vi "ICM Write Characters.vi"(8 "error in (no error)":errorcluster, 9 "Handle In":variant, 10 "Data In":string, 11 "OSDS Format":T1={"Data Stream Name"="", "Version"=0.0, "Author"="", "Reader Name"="", "Parser Name"="", "Description"="", "Comments"="", "Location"="", "Format String"="", "Frame Time"=0, "# of Channels"=0, "# of Records"=0, "Char/Record"=0, "Termination String\nor NTP IP"="", "Bus"=enum."Serial Port", "Port"=1, "Baud Rate"=9600, "Data Bits"=8, "Parity"=enum."None", "Stop Bits"=10, "Flow Control"=0, "Channel Names"=[], "Enabled"=[], "Initialization String"="", "Query String"="", "Reserved String"="", "Reserved Number"=0.0, "Date"=0.0, "Start Time"=0.0} {"Flow Control" items=["None", "XON/XOFF", "RTS/CTS", "XON/XOFF & RTS/CTS", "DTR/DSR", "XON/XOFF & DTR/DSR"]; "Stop Bits" items=["1.0"=10, "1.5"=15, "2.0"=20]; "Data Bits" min=5 max=8 step=1; "Start Time" format="%<%H:%M:%S>t"; "Date" format="%<%Y/%m/%d>T"; "Version" format="%.1g"}) -> (0 "error out":errorcluster, 2 "Bytes Written":i32)   [LabVIEW 2018]
doc: "OSDS Write Characters.vi\n\n This VI is used to write a frame of Siimulated or Play Back data to a communication port.\n\nOCC Streaming Data System Version 1.0\nJune, 2007 Original Code Consulting David Thomson\n www.originalcode.com"
uses:
  MICAS-X/Resources/OSDS/OSDS Subvis/OSDS Format.ctl
  MICAS-X/Resources/OSDS/OSDS Subvis/OSDS Bus.ctl
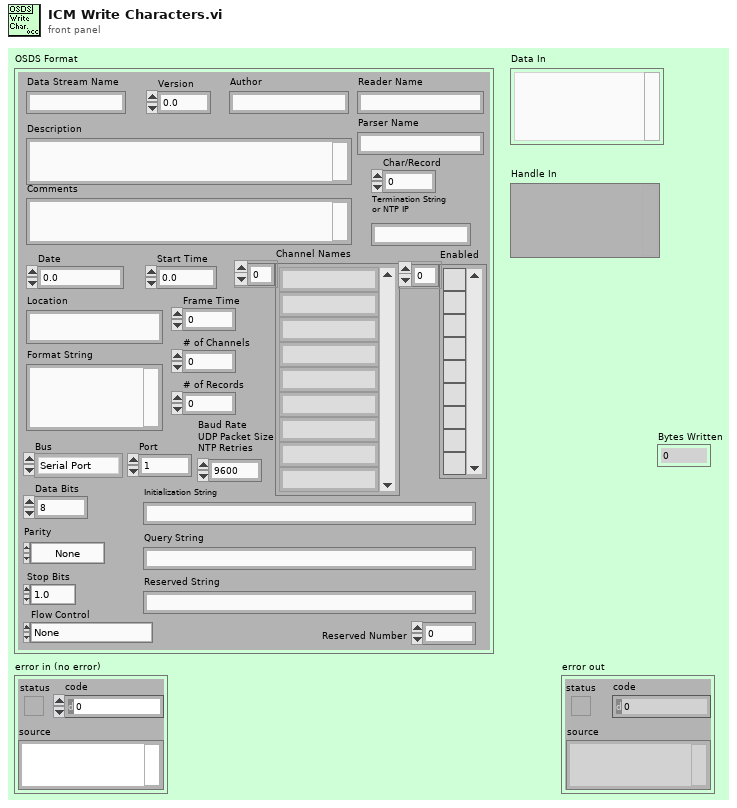
[diagram p1: front panel]
types:
  T1 = typedef "OSDS Format.ctl" = cluster{"Data Stream Name":string, "Version":sgl, "Author":string, "Reader Name":string, "Parser Name":string, "Description":string, "Comments":string, "Location":string, "Format String":string, "Frame Time":i32, "# of Channels":i32, "# of Records":i32, "Char/Record":i32, "Termination String\nor NTP IP":string, "Bus":T2, "Port":i32, "Baud Rate":u32, "Data Bits":u16, "Parity":enum16{"None", "Odd", "Even", "Mark", "Space"}, "Stop Bits":u16, "Flow Control":u16, "Channel Names":string[], "Enabled":bool[], "Initialization String":string, "Query String":string, "Reserved String":string, "Reserved Number":dbl, "Date":dbl, "Start Time":dbl}
  T2 = typedef "OSDS Bus.ctl" = enum16{"Serial Port", "UDP", "NTP", "Local Time", "UTC Time", "UDP MC", "TCP"}
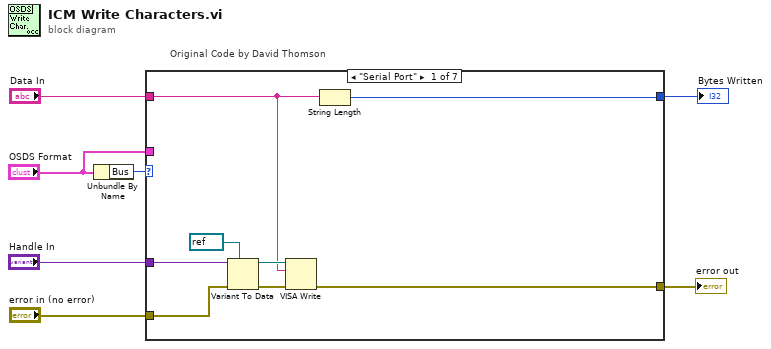
[diagram p0: block diagram]
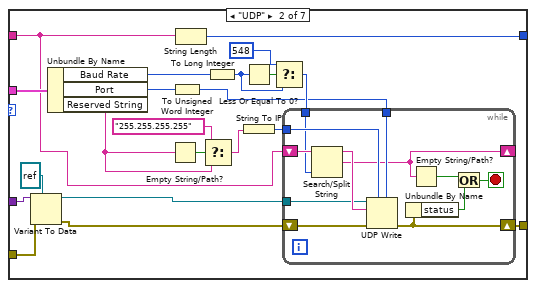
[diagram p2: hidden frame]
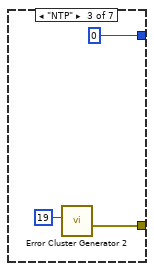
[diagram p3: hidden frame]
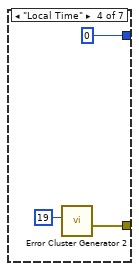
[diagram p4: hidden frame]
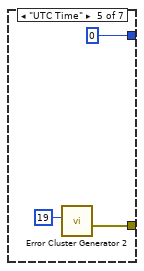
[diagram p5: hidden frame]
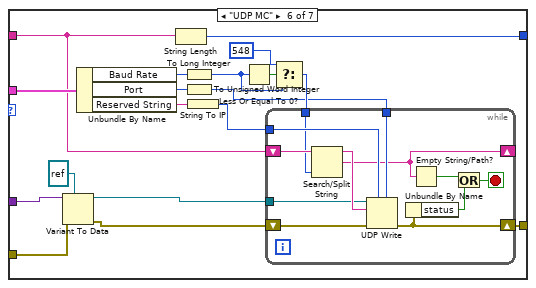
[diagram p6: hidden frame]
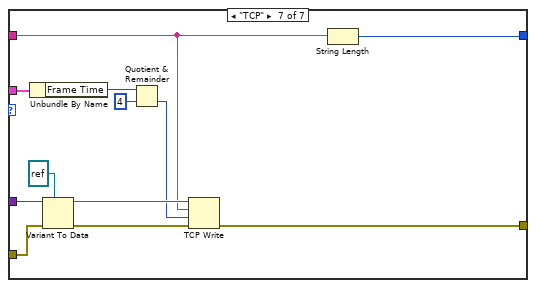
[diagram p7: hidden frame]
diagram:
  n1 = Unbundle By Name("OSDS Format") -> ("Bus"=w7:T2)
  n2 = case "Original Code by David Thomson" shown="\"Serial Port\"" w7 {
    tunnel: "Handle In" -> [w15 w36 _ _ _ w75 w99]
    tunnel: [w10 w28 w50 w52 w55 w67 w94] -> w5
    tunnel: "Data In" -> [w9 w18 _ _ _ w65 w93]
    tunnel: [w13 w34 0 0 0 w73 w92] -> w3
    tunnel: "OSDS Format" -> [_ w33 _ _ _ w72 w90]
    tunnel: "error in (no error)" -> [w8 w23 _ _ _ w61 w98]
    frame "Serial Port" {
      n3 = Variant To Data(error in=w8, type=refnum<visa-resource-name> refnum ("VISA resource name"), Variant=w15) -> (data=w12:refnum<visa-resource-name>, error out=w11:errorcluster)
      n4 = VISA Write(VISA resource name=w12, write buffer=w9, error in (no error)=w11) -> (error out=w10:errorcluster)  [unwired: 2 out]
      n5 = String Length(string=w9) -> (length=w13:i32)
    }
    frame "UDP" {
      n6 = Variant To Data(error in=w23, type=refnum<k16> refnum ("connection ID"), Variant=w36) -> (data=w24:refnum<k16>, error out=w27:errorcluster)
      n7 = Unbundle By Name(w33) -> ("Baud Rate"=w29:u32, "Port"=w26:i32, "Reserved String"=w16:string)
      n8 = Empty String/Path?(string/path=w16) -> (empty?=w20:bool)
      n9 = To Unsigned Word Integer(number=w26) -> (unsigned 16bit integer=w21:u16)
      n10 = String Length(string=w18) -> (length=w34:i32)
      n11 = Select(t="255.255.255.255", s=w20, f=w16) -> (s? t:f=w17:string)
      n12 = To Long Integer(number=w29) -> (32bit integer=w30:i32)
      n13 = Less Or Equal To 0?(x=w30) -> (x <= 0?=w32:bool)
      n14 = String To IP(1:w17) -> (0:w22:u32)
      n15 = Select(t=548 ("max size (548)"), s=w32, f=w30) -> (s? t:f=w25:i32)
      n16 = while {
        shift-right: [w41] -> _
        shift-left: w18 -> [w45]
        shift-right: [w39] -> w28
        shift-left: w27 -> [w48]
        tunnel: w22 -> [w47]
        tunnel: w21 -> [w46]
        tunnel: w25 -> [w44]
        tunnel: w24 -> [w42]
        stop <- w37 stop-if-true
        n17 = Search/Split String(string=w45, offset (0)=w44) -> (substring before match=w43:string, match + rest of string=w41:string)  [unwired: 1 in, 1 out]
        n18 = UDP Write(address=w47, port or service name=w46, connection ID=w42, data in=w43, 8:w48) -> (error out=w39:errorcluster)  [unwired: 2 out]
        n19 = Unbundle By Name(w39) -> ("status"=w38:bool)
        n20 = Empty String/Path?(string/path=w41) -> (empty?=w40:bool)
        n21 = Or(x=w40, y=w38) -> (x .or. y?=w37:bool)
      }
    }
    frame "NTP" {
      n22 = call "Error Cluster Generator 2.vi"("code"=19) -> ("error out"=w50:errorcluster)  [unwired: 3 in, 3 out]
    }
    frame "Local Time" {
      n23 = call "Error Cluster Generator 2.vi"("code"=19) -> ("error out"=w52:errorcluster)  [unwired: 3 in, 3 out]
    }
    frame "UTC Time" {
      n24 = call "Error Cluster Generator 2.vi"("code"=19) -> ("error out"=w55:errorcluster)  [unwired: 3 in, 3 out]
    }
    frame "UDP MC" {
      n25 = Variant To Data(error in=w61, type=refnum<k16> refnum ("connection ID"), Variant=w75) -> (data=w62:refnum<k16>, error out=w66:errorcluster)
      n26 = Unbundle By Name(w72) -> ("Baud Rate"=w68:u32, "Port"=w64:i32, "Reserved String"=w59:string)
      n27 = String Length(string=w65) -> (length=w73:i32)
      n28 = To Long Integer(number=w68) -> (32bit integer=w69:i32)
      n29 = To Unsigned Word Integer(number=w64) -> (unsigned 16bit integer=w60:u16)
      n30 = String To IP(1:w59) -> (0:w58:u32)
      n31 = Less Or Equal To 0?(x=w69) -> (x <= 0?=w71:bool)
      n32 = Select(t=548 ("max size (548)"), s=w71, f=w69) -> (s? t:f=w63:i32)
      n33 = while {
        shift-right: [w80] -> _
        shift-left: w65 -> [w84]
        shift-right: [w78] -> w67
        shift-left: w66 -> [w87]
        tunnel: w58 -> [w86]
        tunnel: w60 -> [w85]
        tunnel: w63 -> [w83]
        tunnel: w62 -> [w81]
        stop <- w76 stop-if-true
        n34 = Search/Split String(string=w84, offset (0)=w83) -> (substring before match=w82:string, match + rest of string=w80:string)  [unwired: 1 in, 1 out]
        n35 = UDP Write(address=w86, port or service name=w85, connection ID=w81, data in=w82, 8:w87) -> (error out=w78:errorcluster)  [unwired: 2 out]
        n36 = Unbundle By Name(w78) -> ("status"=w77:bool)
        n37 = Empty String/Path?(string/path=w80) -> (empty?=w79:bool)
        n38 = Or(x=w79, y=w77) -> (x .or. y?=w76:bool)
      }
    }
    frame "TCP" {
      n39 = Unbundle By Name(w90) -> ("Frame Time"=w88:i32)
      n40 = Variant To Data(error in=w98, type=refnum<k5> refnum ("TCP Ref"), Variant=w99) -> (data=w96:refnum<k5>, error out=w95:errorcluster)
      n41 = Quotient & Remainder(x=w88, y=4) -> (floor(x/y)=w89:i32)  [unwired: 1 out]
      n42 = TCP Write(connection ID=w96, data in=w93, error in (no error)=w95, 9:w89) -> (error out=w94:errorcluster)  [unwired: 2 out]
      n43 = String Length(string=w93) -> (length=w92:i32)
    }
  }
  "error out" <- w5
  "Bytes Written" <- w3
